vi "Load Config.vi"(8 "error in (no error)":errorcluster, 11 "ValveControlModule in":refnum<class "ValveControlModule.lvclass">) -> (0 "error out":errorcluster, 3 "ValveControlModule out":refnum<class "ValveControlModule.lvclass">)   [LabVIEW 2020, in "VolatusControl.lvlib" / "ValveControlModule.lvclass"]
uses:
  ValveControlModule.lvclass
  ValveControlModule.lvclass/ValveControlModule.ctl
  Volatus/Module/Module.lvclass
  VolatusConfig/VolatusConfigElement/VolatusConfigElement.lvclass
  lv-cdm/CDM-Config/Config Element/Config Element.lvclass
  C:/dev/lv20CE/relink/lv-volatus/Volatus/Module/Module.lvclass
  C:/dev/lv20CE/relink/lv-volatus/VolatusControl/ValveControlModule/ValveControlModule.lvclass
  VolatusConfig/Task/Task.lvclass
  C:/dev/lv20CE/relink/lv-volatus/VolatusConfig/VolatusConfigElement/VolatusConfigElement.lvclass
  C:/dev/lv20CE/relink/lv-volatus/VolatusConfig/Task/Task.lvclass
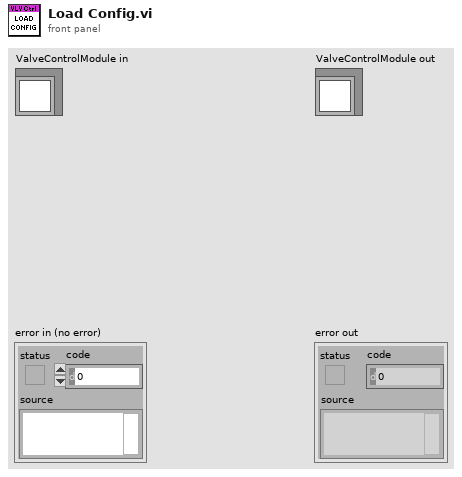
[diagram p1: front panel]
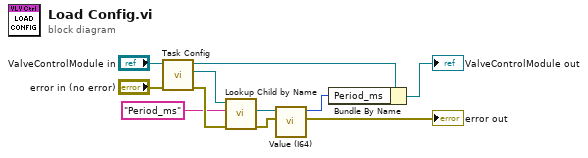
[diagram p0: block diagram]
diagram:
  n1 = call "Task Config.vi"("error in (no error)"="error in (no error)", "Module in"="ValveControlModule in") -> ("error out"=w11:errorcluster, "Task Config"=w7:refnum<class "Task.lvclass">, "Module out"=w8:refnum<class "ValveControlModule.lvclass">)  [unwired: 7 in]
  n2 = call "Lookup Child by Name.vi"("error in (no error)"=w11, "Child Name"="Period_ms", "VolatusConfigElement in"=w7) -> ("error out"=w4:errorcluster, "Child"=w5:refnum<class "Config Element.lvclass">)  [unwired: 5 in, 2 out]
  n3 = call "Value (I64).vi"("error in (no error)"=w4, "Config Element in"=w5) -> ("error out"=→"error out":errorcluster, "I64 Value"=w2:i64)  [unwired: 8 in]
  n4 = Bundle By Name(cluster=w8, "Period_ms"=w2) -> (→"ValveControlModule out":refnum<class "ValveControlModule.lvclass">)
